vi "Obtain Transfer Group.vi"(8 "error in (no error)":errorcluster, 10 "command parameters":T1, 11 "Transceiver Thread in":refnum<class "Plugin Thread.lvclass">) -> (0 "error out":errorcluster, 2 "Transfer Group":refnum<class "Transfer Group.lvclass">, 3 "Transceiver Thread out":refnum<class "Plugin Thread.lvclass">)   [LabVIEW 2021, in "DSF Core.lvlib" / "Plugin Thread.lvclass"]
uses:
  Thread/Plugin/Plugin Thread.lvclass
  Interface/Plugin/Command Parameters.ctl
  Transfer Group/Transfer Group.lvclass
  Thread/Plugin/Plugin Thread.lvclass/Plugin Thread.ctl
  Transfer Group/Transfer Group.lvclass/Transfer Group.ctl
  Timing/Timing.lvclass/Timing.ctl
  Timing/Set Iteration.vi
  Interface/Plugin/Plugin Interface.lvclass
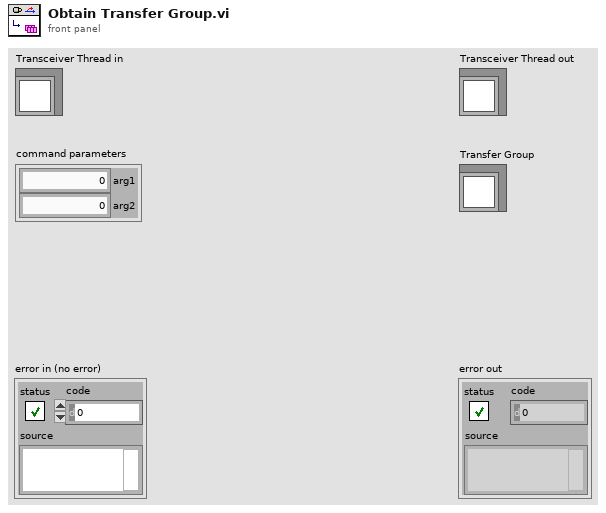
[diagram p1: front panel]
types:
  T1 = typedef "DSF Core.lvlib/Plugin Interface.lvclass/Command Parameters.ctl" = cluster{"arg1":u64, "arg2":u64}
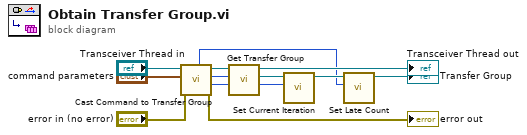
[diagram p0: block diagram]
diagram:
  n1 = call "Cast Command to Transfer Group.vi"("error in (no error)"="error in (no error)", "command parameters"="command parameters", "Plugin Thread in"="Transceiver Thread in") -> ("error out"=→"error out":errorcluster, "Transfer Group iteration"=w1:u64, "Transfer Group id"=w9:u8, "Plugin Thread out"=w10:refnum<class "Plugin Thread.lvclass">, "Transfer Group late count"=w2:i32)  [unwired: 4 in]
  n2 = call "Get Transfer Group.vi"("index"=w9, "Transceiver Thread in"=w10) -> ("Transfer Group"=w7:refnum<class "Transfer Group.lvclass">, "Transceiver Thread out"=→"Transceiver Thread out":refnum<class "Plugin Thread.lvclass">)  [unwired: 8 in]
  n3 = call "Set Current Iteration.vi"("iteration"=w1, "Transfer Group in"=w7) -> ("Transfer Group out"=w4:refnum<class "Transfer Group.lvclass">)  [unwired: 9 in]
  n4 = call "Set Late Count.vi"("late count"=w2, "Transfer Group in"=w4) -> ("Transfer Group out"=→"Transfer Group":refnum<class "Transfer Group.lvclass">)  [unwired: 9 in]
